vi "读取数据.vi"(8 "error in (no error)":errorcluster, 11 "数值类型.lvclass in":refnum<class "数值类型.lvclass">) -> (0 "error out":errorcluster, 2 "数据":dbl, 3 "数值类型.lvclass out":refnum<class "数值类型.lvclass">)   [LabVIEW 2021, in "数值类型.lvclass"]
doc: "本VI是为《我和LabVIEW》一书编写的示例。\n关于本书的介绍请参考网页：\nhttp://ruanqizhen.spaces.live.com/blog/cns!5852D4F797C53FB6!4310.entry"
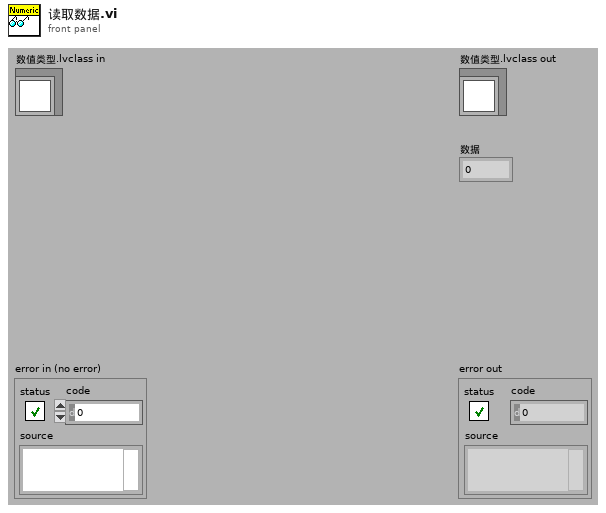
[diagram p1: front panel]
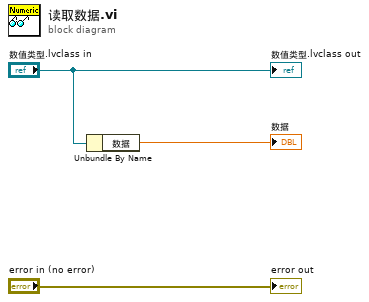
[diagram p0: block diagram]
diagram:
  n1 = Unbundle By Name("数值类型.lvclass in") -> ("数据"=→"数据":dbl)
  "error out" <- "error in (no error)"
  "数值类型.lvclass out" <- "数值类型.lvclass in"
